vi "measure.vi"(10 "Ampiezza":dbl, 11 "Indirizzo Multimetro":string) -> (1 "Vpp=Vout":dbl, 2 "(Vout/Vin)dB":dbl, 3 "Vpp":string, 4 "Vrms=Vin":dbl, 5 "V zero-picco":dbl)   [LabVIEW 2021]
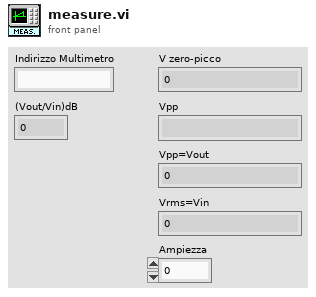
[diagram p1: front panel]
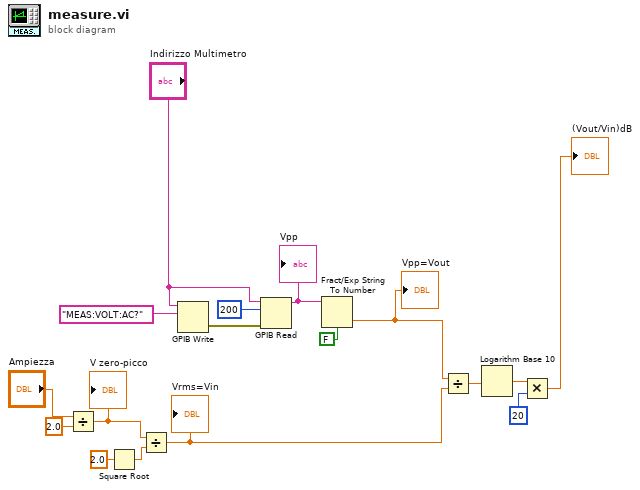
[diagram p0: block diagram]
diagram:
  n1 = Divide(x="Ampiezza", y=2.0) -> (x/y=w9:dbl)
  "V zero-picco" <- w9
  n2 = Square Root(x=2.0) -> (sqrt(x)=w10:dbl)
  n3 = Divide(x=w9, y=w10) -> (x/y=w12:dbl)
  "Vrms=Vin" <- w12
  n4 = GPIB Write(0:"Indirizzo Multimetro", 1:"MEAS:VOLT:AC?" ("data")) -> (6:w2:errorcluster)  [unwired: 3 in, 1 out]
  n5 = GPIB Read(0:"Indirizzo Multimetro", 1:200 ("byte count"), 3:w2) -> (5:w5:string)  [unwired: 2 in, 2 out]
  "Vpp" <- w5
  n6 = Fract/Exp String To Number(use system decimal point (T)=FALSE, string=w5) -> (number=w13:dbl)  [unwired: 2 in, 1 out]
  "Vpp=Vout" <- w13
  n7 = Divide(x=w13, y=w12) -> (x/y=w14:dbl)
  n8 = Logarithm Base 10(1:w14) -> (0:w15:dbl)
  n9 = Multiply(x=w15, y=u32 20) -> (x*y=→"(Vout/Vin)dB":dbl)
